vi "Run.vi"(8 "error in (no error)":errorcluster, 11 "VMR Server in":refnum<class "VMR Server.lvclass">) -> (0 "error out":errorcluster, 3 "VMR Server out":refnum<class "VMR Server.lvclass">)   [LabVIEW 2022 SP3, in "VMR Server.lvlib" / "VMR Server.lvclass"]
uses:
  VMR Server.lvclass
  VMR Server.lvclass/VMR Server.ctl
  <vilib>/IlluminatedG/IG HTTP Server/HTTP Server/Server/Server.lvclass
panel:
  # "VMR Server App"
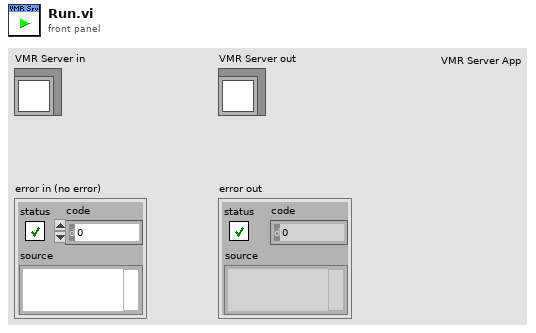
[diagram p1: front panel]
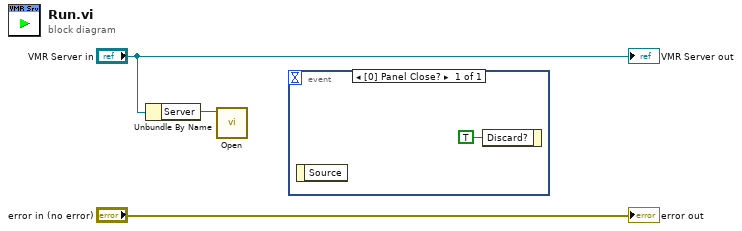
[diagram p0: block diagram]
diagram:
  n1 = Unbundle By Name("VMR Server in") -> ("Server"=w1:refnum<class "Server.lvclass">)
  n2 = call <vilib>:"Open.vi"("Server in"=w1) -> ()  [unwired: 9 in, 2 out]
  n3 = event shown="[0] Panel Close?" {
    selector: _ -> [_]
    dyn-events: _ -> [_]
    timeout: _ -> [_]
    event Panel Close? {
      n4 = event-data() -> ()  [unwired: 1 in, 1 out]
      n5 = event-data("Discard?"=TRUE) -> ()  [unwired: 1 in, 1 out]
    }
  }
  "error out" <- "error in (no error)"
  "VMR Server out" <- "VMR Server in"
